vi "Sprach Index.vi"() -> (3 "Sprache":u16)   [LabVIEW 2015, in "Sprachverwaltung.lvlib"]
uses:
  Sprachverwaltung.lvlib
  <vilib>/Utility/config.llb/Read Key (U32).vi
  <vilib>/Utility/config.llb/NI_LVConfig.lvlib
  Allgemein/allgemeine Sub-VIs.lvlib
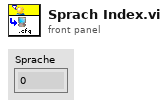
[diagram p1: front panel]
types:
  T1 = typedef "NI_LVConfig.lvlib/Config Data RefNum.ctl" = refnum<k1>
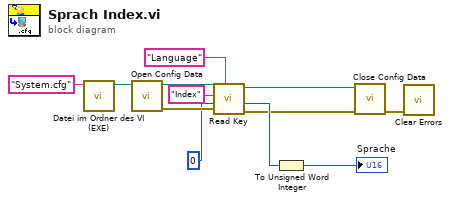
[diagram p0: block diagram]
diagram:
  n1 = call "Datei im Ordner des VI (EXE).vi"("Dateiname"="System.cfg") -> ("Dateipfad im Ordner des Haupt-VIs"=w12:path)  [unwired: 8 in, 2 out]
  n2 = call <vilib>:"Open Config Data.vi"("configuration file path"=w12) -> ("error out"=w7:errorcluster, "refnum"=w3:T1)  [unwired: 8 in, 1 out]
  n3 = call-poly <vilib>:"Read Key.vi"("section"="Language", "error in (no error)"=w7, "default value"=u32 0, "key"="Index", "refnum"=w3) -> ("error out"=w8:errorcluster, "value"=w9:u32, "refnum out"=w10:T1)  [unwired: 3 in, 1 out]
  n4 = To Unsigned Word Integer(number=w9) -> (unsigned 16bit integer=→"Sprache":u16)
  n5 = call <vilib>:"Close Config Data.vi"("error in (no error)"=w8, "refnum"=w10) -> ("error out"=w6:errorcluster)  [unwired: 8 in, 1 out]
  n6 = call <vilib>:"Clear Errors.vi"("error in (no error)"=w6) -> ()  [unwired: 5 in, 2 out]
